vi "Get Registration ID of endpoint.vi"(10 "Endpoint URI":string, 11 "Message loop data (in)":T1) -> (0 "error out":errorcluster, 2 "Registrtion ID":u64, 3 "Message loop data (out)":T1)   [LabVIEW 2020, in "wamplv.lvlib" / "WAMP Client.lvclass"]
uses:
  WAMP Client.lvclass
  WAMP Client.lvclass/WAMP Client.ctl
  <vilib>/ErrorRing/Error Ring.xnode
  <vilib>/Utility/error.llb/Error Cluster From Error Code.vi
  API/TypeDefs/WAMP error (JSON).ctl
  wamplv.lvlib
  API/TypeDefs/Combined error.ctl
  TypeDef/Success or error (JSON).ctl
  TypeDef/Publish Requests Map.ctl
  TypeDef/Endpoint Data.ctl
  TypeDef/CALL Request Map.ctl
  TypeDef/SUBSCRIBE Requests Map.ctl
  TypeDef/Subscriptions Map.ctl
  TypeDef/Unsubscribe Requests Map.ctl
  TypeDef/Unregister request (JSON).ctl
  TypeDef/Unregister requests map.ctl
  TypeDef/Message Loop Data.ctl
  Private/Requests/Call/ICallRequest/ICallRequest.lvclass
  Private/Requests/Subscribe/ISubscribe/ISubscribe.lvclass
  Private/Requests/Publish/IPublish/IPublish.lvclass
  Private/Message loop classes/Subscription details/SubscriptionDetailsParent/SubscriptionDetailsParent.lvclass
  Private/Requests/Unsubscribe/IUnsubscribe/IUnsubscribe.lvclass
  Private/Requests/Register/IRegister/IRegister.lvclass
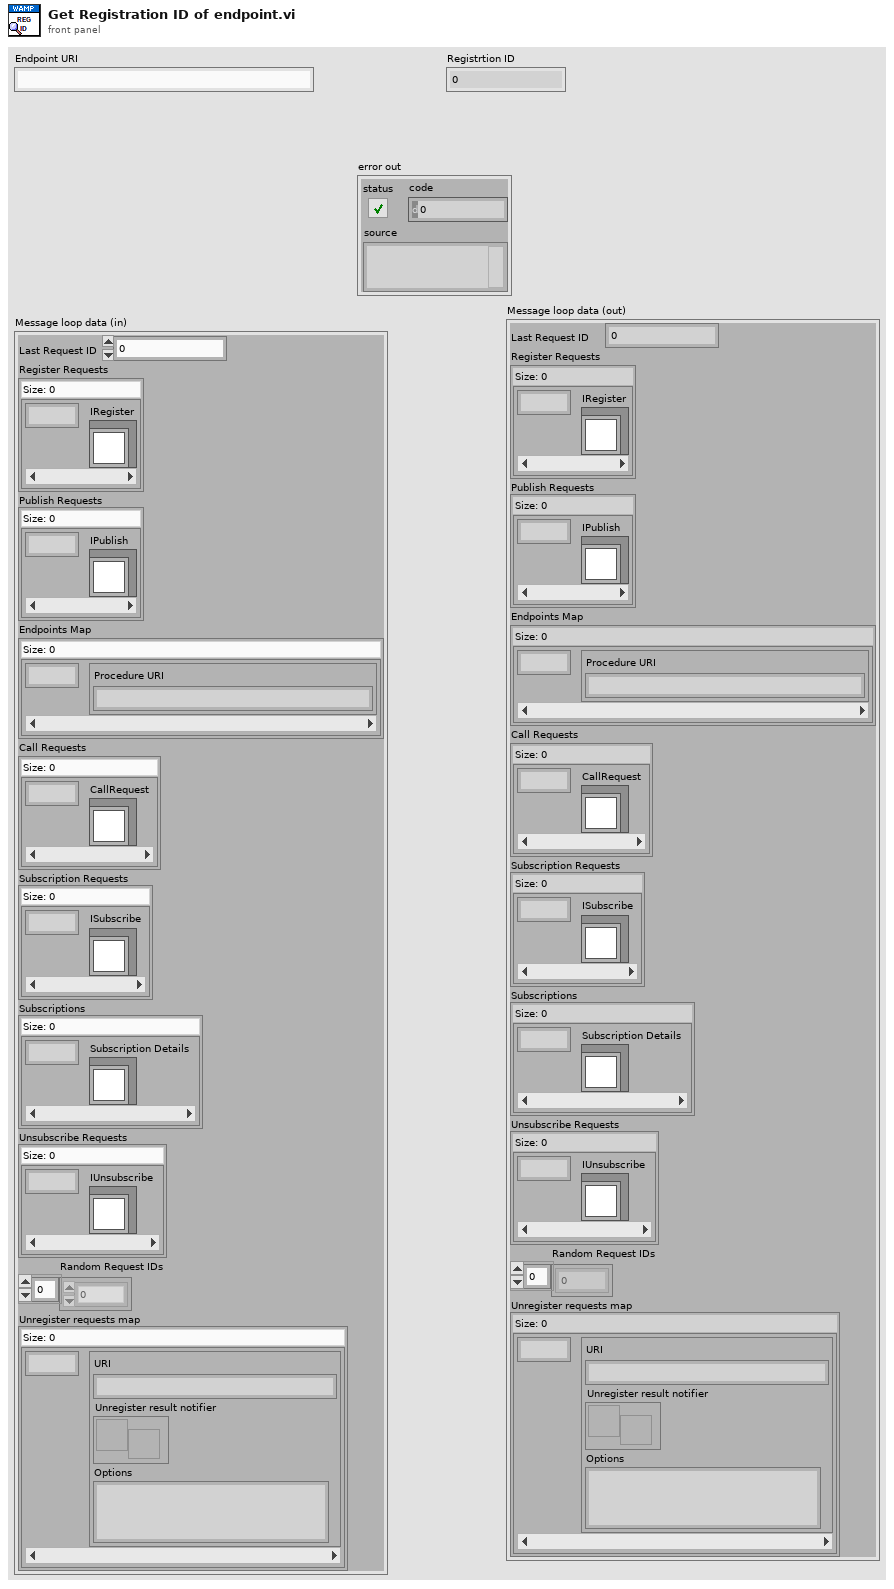
[diagram p1: front panel]
types:
  T1 = typedef "wamplv.lvlib/Message Loop Data.ctl" = cluster{"Last Request ID":u64, "Register Requests":map{u64, refnum<class "IRegister.lvclass">}, "Publish Requests":T2, "Endpoints Map":map{u64, T3}, "Call Requests":T4, "Subscription Requests":T5, "Subscriptions":T6, "Unsubscribe Requests":T7, "Random Request IDs":u64[], "Unregister requests map":T8}
  T2 = typedef "wamplv.lvlib/Publish Requests Map.ctl" = map{u64, refnum<class "IPublish.lvclass">}
  T3 = typedef "wamplv.lvlib/Endpoint Data.ctl" = cluster{"Procedure URI":string}
  T4 = typedef "wamplv.lvlib/CALL Request Map.ctl" = map{u64, refnum<class "ICallRequest.lvclass">}
  T5 = typedef "wamplv.lvlib/SUBSCRIBE Requests Map.ctl" = map{u64, refnum<class "ISubscribe.lvclass">}
  T6 = typedef "wamplv.lvlib/Subscriptions Map.ctl" = map{u64, refnum<class "SubscriptionDetailsParent.lvclass">}
  T7 = typedef "wamplv.lvlib/Unsubscribe Requests Map.ctl" = map{u64, refnum<class "IUnsubscribe.lvclass">}
  T8 = typedef "wamplv.lvlib/Unregister requests map.ctl" = map{u64, T9}
  T9 = typedef "wamplv.lvlib/Unregister request (JSON).ctl" = cluster{"URI":string, "Unregister result notifier":refnum<notifier>, "Options":string}
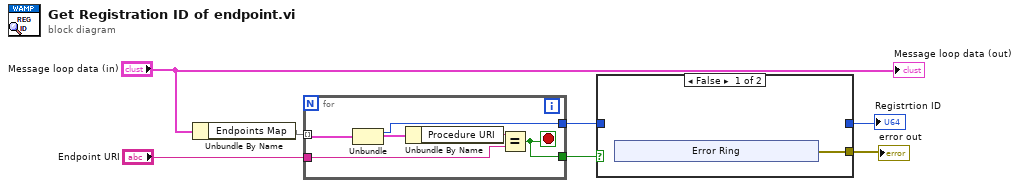
[diagram p0: block diagram]
diagram:
  n1 = Unbundle By Name("Message loop data (in)") -> ("Endpoints Map"=w5:map{u64, T3})
  n2 = for {
    tunnel: w5 -> [w13] mode=indexing
    tunnel: "Endpoint URI" -> [w9]
    tunnel: [w11] -> w3
    tunnel: [w8] -> w4
    stop <- w8 stop-if-true
    n3 = Unbundle(w13) -> ("key"=w11:u64, "Endpoint Data"=w12:T3)
    n4 = Unbundle By Name(w12) -> ("Procedure URI"=w10:string)
    n5 = Equal?(x=w10, y=w9) -> (x = y?=w8:bool)
  }
  n6 = case shown="False" w4 {
    tunnel: w3 -> [_ w19]
    tunnel: [_ w19] -> w2
    tunnel: [w14 _] -> w1
    frame False {
      n7 = xnode "Error Ring"() -> ("error out"=w14:errorcluster)
    }
    frame True {
    }
  }
  "Registrtion ID" <- w2
  "error out" <- w1
  "Message loop data (out)" <- "Message loop data (in)"
